vi "test_CRIO RTD.vi"() -> ()   [LabVIEW 2023]
uses:
  Measure and Stimulus Subsystems/Measure and Stimulus Subsystems.lvclass
  Thermometer DAQmx RTD Cont CFG.lvclass
  Virt Instr Host/Virt Instr Local.lvclass
panel:
  out "error out":errorcluster
  in  "Error In":errorcluster
  out "Output":variant
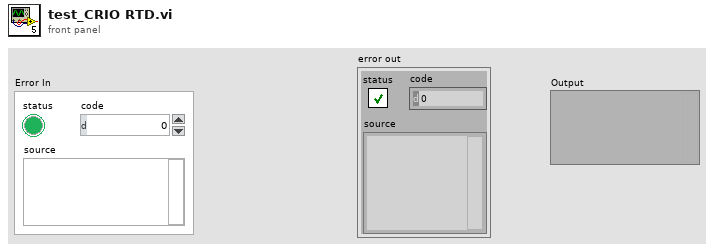
[diagram p1: front panel]
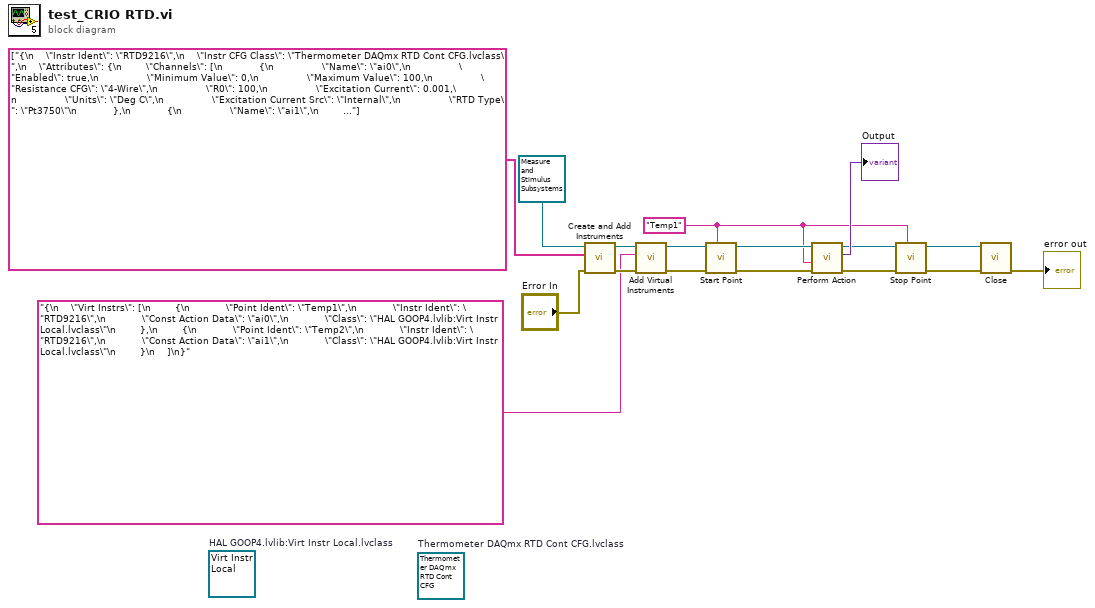
[diagram p0: block diagram]
diagram:
  w1 = "Temp1" ("Point Ident")
  (unwired) refnum<class "Virt Instr Local.lvclass"> refnum  # HAL GOOP4.lvlib:Virt Instr Local.lvclass
  (unwired) refnum<class "Thermometer DAQmx RTD Cont CFG.lvclass"> refnum  # Thermometer DAQmx RTD Cont CFG.lvclass
  n1 = call "Create and Add Instruments.vi"("Error In"="Error In", "Physical Intr CFGs"=string[] ["{\n    \"Instr Ident\": \"RTD9216\",\n    \"Instr CFG Class\": \"Thermometer DAQmx RTD Cont CFG.lvclass\",\n    \"Attributes\": {\n        \"Channels\": [\n            {\n                \"Name\": \"ai0\",\n                \"Enabled\": true,\n                \"Minimum Value\": 0,\n                \"Maximum Value\": 100,\n                \"Resistance CFG\": \"4-Wire\",\n                \"R0\": 100,\n                \"Excitation Current\": 0.001,\n                \"Units\": \"Deg C\",\n                \"Excitation Current Src\": \"Internal\",\n                \"RTD Type\": \"Pt3750\"\n            },\n            {\n                \"Name\": \"ai1\",\n                \"Enabled\": true,\n                \"Minimum Value\": 0,\n                \"Maximum Value\": 100,\n                \"Resistance CFG\": \"3-Wire\",\n                \"R0\": 100,\n                \"Excitation Current\": 0.001,\n                \"Units\": \"Deg C\",\n                \"Excitation Current Src\": \"Internal\",\n                \"RTD Type\": \"Pt3750\"\n            },\n            {\n                \"Name\": \"ai2\",\n                \"Enabled\": false,\n                \"Minimum Value\": 0,\n                \"Maximum Value\": 100,\n                \"Resistance CFG\": \"4-Wire\",\n                \"R0\": 100,\n                \"Excitation Current\": 0.001,\n                \"Units\": \"Deg C\",\n                \"Excitation Current Src\": \"Internal\",\n                \"RTD Type\": \"Pt3750\"\n            }\n        ],\n        \"Timing\": {\n            \"Type\": \"Sample Clock\",\n            \"Samples per Channel\": 1000,\n            \"Sample Mode\": \"Continuous Samples\",\n            \"Sample Rate\": 10,\n            \"Sample Clock Source\": \"OnboardClock\",\n            \"Active Edge\": \"Rising\"\n        },\n        \"Trigger\": {\n            \"Trigger Type\": \"No Trigger\"\n        }\n    }\n}"], "MSS in"=refnum<class "Measure and Stimulus Subsystems.lvclass"> refnum) -> ("Error Out"=w15:errorcluster, "MSS out"=w14:refnum<class "Measure and Stimulus Subsystems.lvclass">)  [unwired: 7 in]
  n2 = call "Add Virtual Instruments.vi"("error in"=w15, "<JSON CFG>"="{\n    \"Virt Instrs\": [\n        {\n            \"Point Ident\": \"Temp1\",\n            \"Instr Ident\": \"RTD9216\",\n            \"Const Action Data\": \"ai0\",\n            \"Class\": \"HAL GOOP4.lvlib:Virt Instr Local.lvclass\"\n        },\n        {\n            \"Point Ident\": \"Temp2\",\n            \"Instr Ident\": \"RTD9216\",\n            \"Const Action Data\": \"ai1\",\n            \"Class\": \"HAL GOOP4.lvlib:Virt Instr Local.lvclass\"\n        }\n    ]\n}", "MSS in"=w14) -> ("error out"=w12:errorcluster, "MSS out"=w6:refnum<class "Measure and Stimulus Subsystems.lvclass">)  [unwired: 7 in]
  n3 = call "Start Point.vi"("Point Ident"=w1, "error in"=w12, "MSS in"=w6) -> ("error out"=w7:errorcluster, "MSS out"=w5:refnum<class "Measure and Stimulus Subsystems.lvclass">)  [unwired: 7 in]
  n4 = call "Perform Action.vi"("error in"=w7, "Point Ident"=w1, "MSS in"=w5) -> ("error out"=w11:errorcluster, "Output"=→"Output":variant, "MSS out"=w3:refnum<class "Measure and Stimulus Subsystems.lvclass">)  [unwired: 6 in]
  n5 = call "Stop Point.vi"("Point Ident"=w1, "error in"=w11, "MSS in"=w3) -> ("error out"=w4:errorcluster, "MSS out"=w2:refnum<class "Measure and Stimulus Subsystems.lvclass">)  [unwired: 7 in]
  n6 = call "Close.vi"("error in"=w4, "MSS in"=w2) -> ("error out"=→"error out":errorcluster)  [unwired: 8 in, 1 out]
